vi "RegAllErrorEvents.vi"(8 "ErrorIn":errorcluster[](array[cluster]), 11 "Test.lvclass":refnum<class "Test.lvclass">) -> (0 "ErrorOut":errorcluster[](array[cluster]), 2 "Event Registration Refnum":refnum<event-registration>, 3 "Test.lvclass":refnum<class "Test.lvclass">)   [LabVIEW 2018, in "Test.lvclass"]
uses:
  Test.lvclass
  Sync/SyncModule/Protected/clEventType.ctl
  Digitizer/DigitizerShared/clEventType.ctl
  FGen/FgenShared/clEventType.ctl
  Scope/ScopeShared/clEventType.ctl
  Sensor/SensorShared/clEventType.ctl
  AcPwr/AcPwrShared/clEventType.ctl
  Test.lvclass/Test.ctl
  Accessors/Read ErrorSeverity.vi
  <userlib>/NIST/NISTErrorLib/NISTErrorLib.lvlib
  Sync/SyncModule/SyncModule.lvlib
  Digitizer/DigitizerModule/DigitizerModule.lvlib
  Scope/ScopeModule/ScopeModule.lvlib
  Analysis/AnalysisModule/AnalysisModule.lvlib
  Sensor/SensorModule/SensorModule.lvlib
  AcPwr/AcPwrShared/AcPwrShared.lvlib
  FGen/FgenShared/FgenShared.lvlib
  Sensor/SensorShared/SensorShared.lvlib
  Scope/ScopeShared/ScopeShared.lvlib
  Digitizer/DigitizerShared/DigitizerShared.lvlib
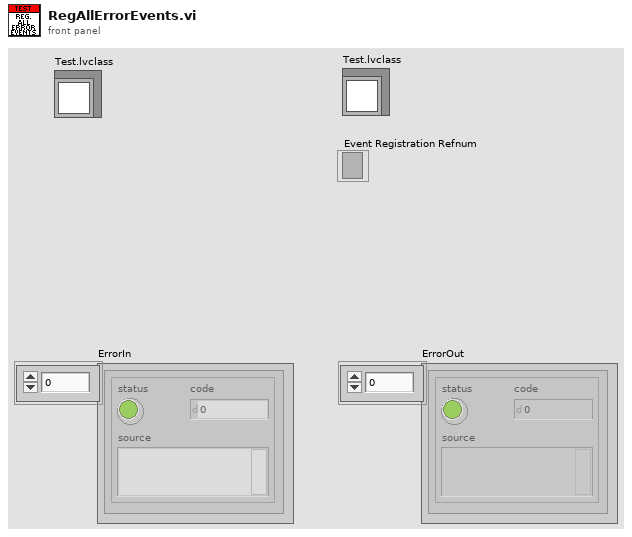
[diagram p1: front panel]
types:
  T1 = typedef "SyncModule.lvlib/SyncBroadcastEvents.ctl" = cluster{"DidInit":refnum<user-event>, "StatusUpdate":refnum<user-event>, "ErrorReport":refnum<user-event>, "DidStop":refnum<user-event>, "PathToINI":refnum<user-event>, "TriggerTime":refnum<user-event>, "LockStatus":refnum<user-event>, "Info":refnum<user-event>, "ClockProperties":refnum<user-event>, "SyncData":refnum<user-event>, "TimingSession":refnum<user-event>}
  T2 = typedef "DigitizerShared.lvlib/clBroadcastEvents.ctl" = cluster{"DidInit":refnum<user-event>, "StatusUpdate":refnum<user-event>, "ErrorReport":refnum<user-event>, "DidStop":refnum<user-event>, "PathToINI":refnum<user-event>, "Channels":refnum<user-event>, "Acq":refnum<user-event>, "Trigger":refnum<user-event>, "Waveforms":refnum<user-event>}
  T3 = typedef "FgenShared.lvlib/clBroadcastEvents.ctl" = cluster{"DidInit":refnum<user-event>, "StatusUpdate":refnum<user-event>, "ErrorReport":refnum<user-event>, "DidStop":refnum<user-event>, "PathToINI":refnum<user-event>, "Channels":refnum<user-event>, "Function":refnum<user-event>, "Waveforms":refnum<user-event>, "Triggers":refnum<user-event>, "FunctionParams":refnum<user-event>, "FunctionArbs":refnum<user-event>, "FunctionSampleRate":refnum<user-event>}
  T4 = typedef "ScopeShared.lvlib/clBroadcastEvents.ctl" = cluster{"DidInit":refnum<user-event>, "StatusUpdate":refnum<user-event>, "ErrorReport":refnum<user-event>, "DidStop":refnum<user-event>, "PathToINI":refnum<user-event>, "Handle":refnum<user-event>, "Model":refnum<user-event>, "Channels":refnum<user-event>, "Acquisition":refnum<user-event>, "Trigger":refnum<user-event>, "ExtAcquisition":refnum<user-event>, "Waveform":refnum<user-event>}
  T5 = typedef "SensorShared.lvlib/clBroadcastEvents.ctl" = cluster{"DidInit":refnum<user-event>, "StatusUpdate":refnum<user-event>, "ErrorReport":refnum<user-event>, "DidStop":refnum<user-event>, "PathToINI":refnum<user-event>, "SensorReport":refnum<user-event>, "SensorConfig":refnum<user-event>}
  T6 = typedef "AcPwrShared.lvlib/AcPwrBroadcastEvents.ctl" = cluster{"DidInit":refnum<user-event>, "StatusUpdate":refnum<user-event>, "ErrorReport":refnum<user-event>, "DidStop":refnum<user-event>, "PathToINI":refnum<user-event>, "Measurements":refnum<user-event>, "LoadConfigFile":refnum<user-event>, "GetSettings":refnum<user-event>, "SetSettings":refnum<user-event>, "GetType&ID":refnum<user-event>, "GotSettings":refnum<user-event>, "GotSettingsLV":refnum<user-event>}
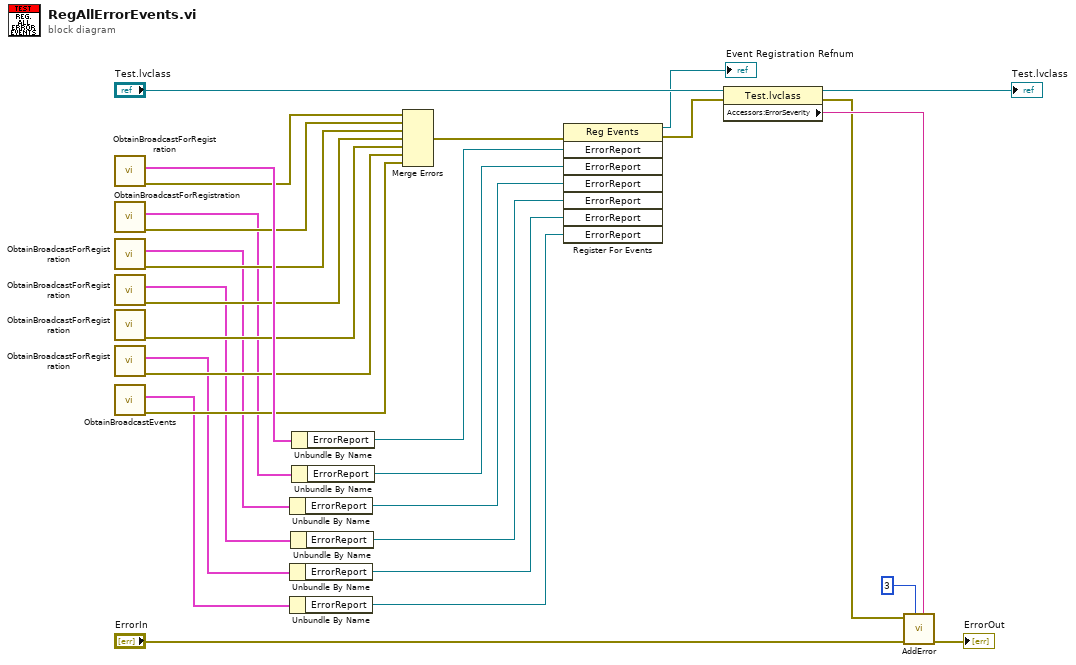
[diagram p0: block diagram]
diagram:
  n1 = call "ObtainBroadcastForRegistration.vi"() -> ("error out"=w18:errorcluster, "SyncBroadcastEvents"=w22:T1)  [unwired: 10 in]
  n2 = call "ObtainBroadcastForRegistration.vi"() -> ("error out"=w17:errorcluster, "clDigitizerBdcstEvents"=w11:T2)  [unwired: 10 in]
  n3 = call "ObtainBroadcastForRegistration.vi"() -> ("error out"=w16:errorcluster, "FgenBroadcastEvents"=w9:T3)  [unwired: 10 in]
  n4 = call "ObtainBroadcastForRegistration.vi"() -> ("error out"=w15:errorcluster, "ScopeBroadcastEvents"=w7:T4)  [unwired: 10 in]
  n5 = call "ObtainBroadcastForRegistration.vi"() -> ("error out"=w14:errorcluster)  [unwired: 10 in, 1 out]
  n6 = call "ObtainBroadcastForRegistration.vi"() -> ("error out"=w13:errorcluster, "SensorBdcstEvents"=w5:T5)  [unwired: 10 in]
  n7 = call "ObtainBroadcastEvents.vi"() -> ("error out"=w12:errorcluster, "AcPwrEvents"=w3:T6)  [unwired: 10 in]
  n8 = Unbundle By Name(w9) -> ("ErrorReport"=w8:refnum<user-event>)
  n9 = Unbundle By Name(w5) -> ("ErrorReport"=w4:refnum<user-event>)
  n10 = Unbundle By Name(w3) -> ("ErrorReport"=w2:refnum<user-event>)
  n11 = Unbundle By Name(w7) -> ("ErrorReport"=w6:refnum<user-event>)
  n12 = Unbundle By Name(w22) -> ("ErrorReport"=w21:refnum<user-event>)
  n13 = Unbundle By Name(w11) -> ("ErrorReport"=w10:refnum<user-event>)
  n14 = Merge Errors(w18, w17, w16, w15, w14, w13, w12) -> (w19:errorcluster)
  n15 = register-events(error in=w19, w21, w10, w8, w6, w4, w2) -> (reference out=→"Event Registration Refnum":refnum<event-registration>, error out=w20:errorcluster)  [unwired: 1 in]
  n16 = property class="Test.lvclass"(reference="Test.lvclass", error in=w20) -> (reference out=→"Test.lvclass":refnum<class "Test.lvclass">, error out=w25:errorcluster, "Accessors:ErrorSeverity"=w27:string)
  n17 = call <userlib>:"AddError.vi"("Severity"=w27, "Priority"=u8 3, "ErrorArray In"="ErrorIn", "error in (no error)"=w25) -> ("ErrorArray Out"=→"ErrorOut":errorcluster[])  [unwired: 6 in, 1 out]
